vi "PH_Trendviewer_Powermeter.export Data.vi"(0 "i ref in":refnum<vi>, 5 "error in (no error)":errorcluster) -> (14 "i ref out":refnum<vi>, 19 "error out":errorcluster)   [LabVIEW 2014, in "PH_Trendviewer_Powermeter.lvlib"]
doc: "This VI exports data to a file"
uses:
  PH_Trendviewer_Powermeter.lvlib
  PH_Common/PH_Common.lvlib
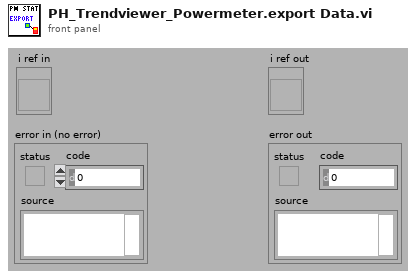
[diagram p1: front panel]
types:
  T1 = typedef "PH_Trendviewer_Powermeter.lvlib/PH_Trendviewer_Powermeter.i attribute.ctl" = cluster{"GUI Refs ":cluster{"Status":refnum<vi>, "Result Graph":refnum<vi>, "Mean Data":refnum<vi>, "Std Dev Data":refnum<vi>, "Dummy Mean":refnum<vi>, "Dummy Std Dev":refnum<vi>, "Export Data":refnum<vi>, "Stat or Trend":refnum<vi>, "Delete":refnum<vi>, "Powermeter":refnum<vi>, "Start":refnum<vi>}, "Powermeter":string, "Stat or Trend":bool, "Start":bool, "Data":cluster{"Time Stamp":timestamp, "Energy [J]":dbl}[], "Datasets strored":i32, "Dataarray Size":i32}
  T2 = cluster{"Time Stamp":timestamp, "Energy [J]":dbl}[]
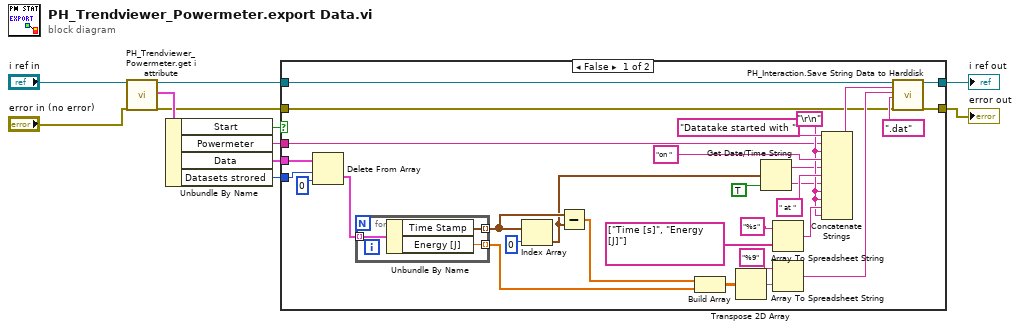
[diagram p0: block diagram]
diagram:
  n1 = call "PH_Trendviewer_Powermeter.get i attribute.vi"("i ref in"="i ref in", "error in (no error)"="error in (no error)") -> ("i ref out"=w5:refnum<vi>, "i attribute"=w9:T1, "error out"=w7:errorcluster)  [unwired: 15 in]
  n2 = Unbundle By Name(w9) -> ("Start"=w6:bool, "Powermeter"=w2:string, "Data"=w3:T2, "Datasets strored"=w1:i32)
  n3 = case shown="False" w6 {
    tunnel: [w41 w46] -> w8
    tunnel: w7 -> [w17 w46]
    tunnel: w5 -> [w18 w45]
    tunnel: [w40 w45] -> w4
    tunnel: w3 -> [w15 _]
    tunnel: w2 -> [w16 _]
    tunnel: w1 -> [w14 _]
    frame False {
      w30 = "\r\n"
      n4 = Delete From Array(array=w15, length=w14, index=0) -> (deleted portion=w13:T2)  [unwired: 1 out]
      n5 = for {
        tunnel: w13 -> [w44] mode=indexing
        tunnel: [w43] -> w39 mode=indexing
        tunnel: [w42] -> w20 mode=indexing
        n6 = Unbundle By Name(w44) -> ("Time Stamp"=w43:timestamp, "Energy [J]"=w42:dbl)
      }
      n7 = Index Array(array=w39, index=0) -> (element=w19:timestamp)
      n8 = Subtract(x=w39, y=w19) -> (x-y=w37:dbl[])
      n9 = Build Array(w37, w20) -> (w28:dbl[][])
      n10 = Transpose 2D Array(2D array=w28) -> (transposed array=w29:dbl[][])
      n11 = Get Date/Time String(seconds (now)=w19, want seconds? (F)=TRUE) -> (date string=w23:string, time string=w22:string)  [unwired: 1 in]
      n12 = Array To Spreadsheet String(array=string[] ["Time [s]", "Energy [J]"], 3:"%s" ("format string")) -> (spreadsheet string=w31:string)  [unwired: 1 in]
      n13 = Array To Spreadsheet String(array=w29, 3:"%9" ("format string")) -> (spreadsheet string=w27:string)  [unwired: 1 in]
      n14 = Concatenate Strings("Datatake started with " ("string"), w16, w30, "on ", w23, " at " ("string"), w22, w30, w30, w31, w30) -> (w25:string)
      n15 = call "PH_Interaction.Save String Data to Harddisk.vi"("i ref in"=w18, "Explanation (for Example: Column 1: xxx, ...)"=w25, "Data (for example: Columns)"=w27, "file name extension"=".dat" ("file name extinction"), "error in (no error)"=w17) -> ("i ref out"=w40:refnum<vi>, "error out"=w41:errorcluster)  [unwired: 12 in, 1 out]
    }
    frame True {
    }
  }
  "error out" <- w8
  "i ref out" <- w4
